vi "Remote Video stream.vi"(1 "Quality":i32=750 min=0 max=1000, 2 "Resolution":T1=1 items=["Low", "Med.", "High", "Max."], 3 "Camera":T2="Travcam") -> (0 "Error out":errorcluster)   [LabVIEW 2016]
uses:
  Camera enum/Camera enum.ctl
  Camera enum/Camera resolution.ctl
  Globals/CamServer global.vi
panel:
  # "PN 21/08/15"
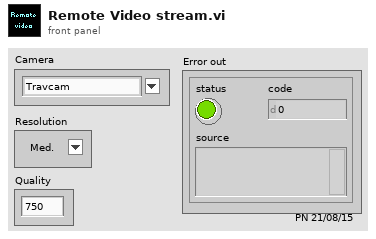
[diagram p1: front panel]
types:
  T1 = typedef "Camera resolution.ctl" = u8
  T2 = typedef "Camera enum.ctl" = string
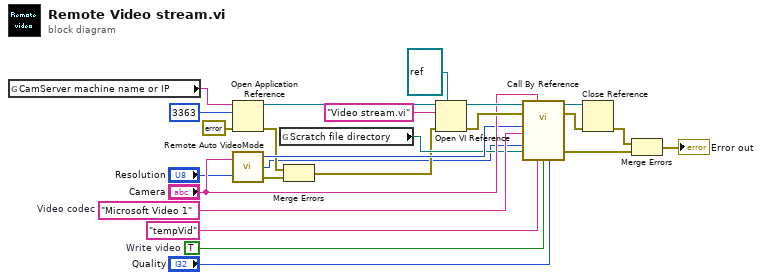
[diagram p0: block diagram]
diagram:
  w9 = "Microsoft Video 1"  # Video codec
  w10 = TRUE  # Write video
  n1 = global read "CamServer global.vi" "CamServer machine name or IP"() -> (w8:string)
  n2 = Open Application Reference(8:errorcluster {"status"=FALSE, "code"=0, "source"=""} ("error in (no error)"), 10:u16 3363 ("port"), 11:w8) -> (0:w6:errorcluster, 3:w23:refnum<vi>)  [unwired: 1 in]
  n3 = call "Remote Auto VideoMode.vi"("Camera"="Camera", "Resolution"="Resolution") -> ("VideoMode"=w13:u32, "FPS"=w1:u32, "Error out"=w5:errorcluster)
  n4 = global read "CamServer global.vi" "Scratch file directory"() -> (w7:path)
  n5 = Merge Errors(w6, w5) -> (w4:errorcluster)
  n6 = Open VI Reference(type specifier VI Refnum (for type only)=refnum<vi> refnum, application reference (local)=w23, vi path="Video stream.vi" ("machine name"), error in (no error)=w4) -> (vi reference=w21:refnum<vi>, error out=w22:errorcluster)  [unwired: 2 in]
  n7 = call-by-ref "?"(reference=w21, error in=w22, "VideoMode"=w13, "Interface name"="Camera", "Video codec"=w9, "FPS"=w1, "Video directory path"=w7, "Video name"="tempVid" ("Image name"), "Write video"=w10, "Quality"="Quality") -> (reference out=w19:refnum<vi>, error out=w18:errorcluster, "Error Out"=w17:errorcluster)  [unwired: 7 in]
  n8 = Close Reference(reference=w19, error in (no error)=w18) -> (error out=w16:errorcluster)
  n9 = Merge Errors(w16, w17) -> (→"Error out":errorcluster)
